vi "setUp.vi"(8 "error in (no error)":errorcluster, 11 "reference in":refnum<class "Scan Engine Scripting API Custom Device Unit Tests.lvclass">) -> (0 "error out":errorcluster, 3 "reference out":refnum<class "Scan Engine Scripting API Custom Device Unit Tests.lvclass">)   [LabVIEW 2019, in "Scan Engine Scripting API Custom Device Unit Tests.lvclass"]
doc: "setUp runs prior to the test method during test execution. Use this method to initialize any object data required by your tests."
uses:
  Scan Engine Scripting API Custom Device Unit Tests.lvclass
  C:/Program Files (x86)/National Instruments/LabVIEW 2019/vi.lib/addons/_JKI Toolkits/VI Tester/TestCase.llb/TestCase.lvclass
  Scan Engine Scripting API Custom Device Unit Tests.lvclass/Scan Engine Scripting API Custom Device Unit Tests.ctl
  <vilib>/addons/_JKI Toolkits/VI Tester/TestCase.llb/TestCase.lvclass
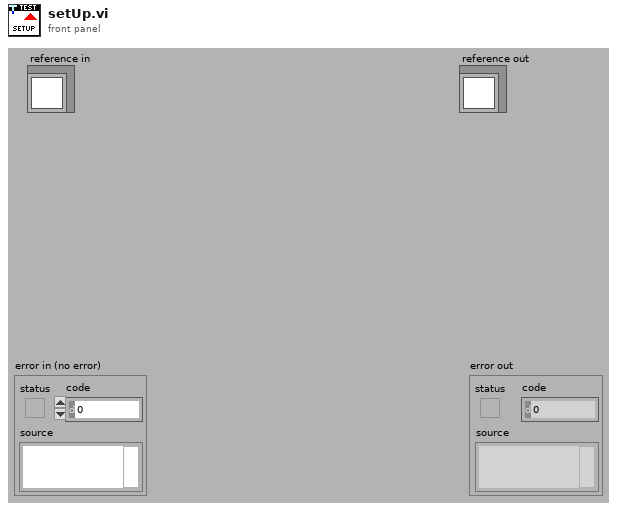
[diagram p1: front panel]
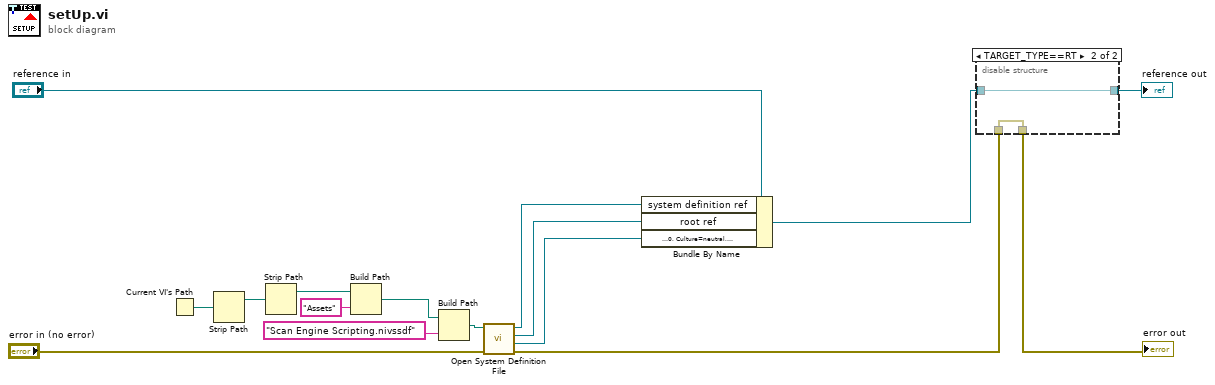
[diagram p0: block diagram]
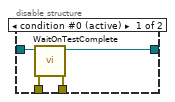
[diagram p2: hidden frame]
diagram:
  n1 = Current VI's Path() -> (path=w12:path)
  n2 = Strip Path(path=w12) -> (stripped path=w11:path)  [unwired: 1 out]
  n3 = Strip Path(path=w11) -> (stripped path=w10:path)  [unwired: 1 out]
  n4 = Build Path(base path=w10, name or relative path="Assets") -> (appended path=w8:path)
  n5 = Build Path(base path=w8, name or relative path="Scan Engine Scripting.nivssdf") -> (appended path=w6:path)
  n6 = call "Open System Definition File.vi"("error in"="error in (no error)", "path"=w6) -> ("error out"=w4:errorcluster, "target ref"=w1:refnum<k24>, "root ref"=w2:refnum<k24>, "system definition ref"=w3:refnum<k24>)  [unwired: 6 in]
  n7 = Bundle By Name(cluster="reference in", "system definition ref"=w3, "root ref"=w2, "target ref"=w1) -> (w13:refnum<class "Scan Engine Scripting API Custom Device Unit Tests.lvclass">)
  n8 = disable-structure shown="TARGET_TYPE==RT" {
    disable-tunnel: w4 -> [w20 w21]
    disable-tunnel: [w19 w21] -> w16
    disable-tunnel: [w18 w22] -> w15
    disable-tunnel: w13 -> [w17 w22]
    frame condition #0 (active) {
      n9 = call <vilib>:"WaitOnTestComplete.vi"("error in (no error)"=w20, "TestCase in"=w17) -> ("error out"=w19:errorcluster, "TestCase out"=w18:refnum<class "Scan Engine Scripting API Custom Device Unit Tests.lvclass">)  [unwired: 8 in]
    }
    frame condition #1 {
    }
  }
  "error out" <- w16
  "reference out" <- w15
